vi "SSL Vision Client.vi"() -> ()   [LabVIEW 2016]
uses:
  <vilib>/Utility/tcp.llb/UDP Multicast Read-Only Open.vi
  SSL Detection Robot.ctl
  SSL Detection Ball.ctl
  SSL Detection Frame.ctl
  SSL Geometry Camera Calibration.ctl
panel:
  out "2D Picture":picture
  out "Geometry Camera Calibration":T1
  out "Field Size":T2
  out "Detection Frame":T3
  out "error out":errorcluster
  out "size(s)":i32
  out "unsigned byte array":u8[](array[numeric]) format="%02x"
  in  "Multicast Address:":string="224.5.23.2"
  in  "Multicast Port:":u16=10020
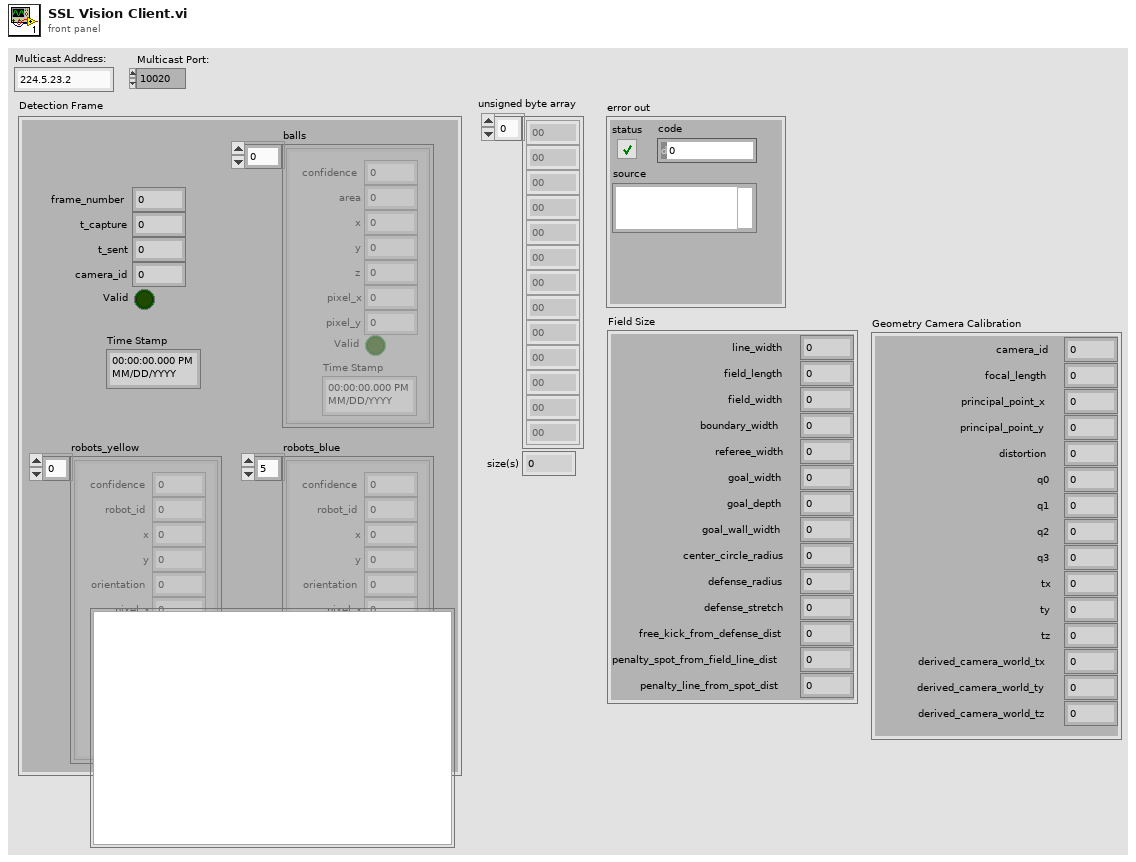
[diagram p1: front panel]
types:
  T1 = typedef "SSL Geometry Camera Calibration.ctl" = cluster{"camera_id":u32, "focal_length":sgl, "principal_point_x":sgl, "principal_point_y":sgl, "distortion":sgl, "q0":sgl, "q1":sgl, "q2":sgl, "q3":sgl, "tx":sgl, "ty":sgl, "tz":sgl, "derived_camera_world_tx":sgl, "derived_camera_world_ty":sgl, "derived_camera_world_tz":sgl}
  T2 = cluster{"line_width":u32, "field_length":u32, "field_width":u32, "boundary_width":u32, "referee_width":u32, "goal_width":u32, "goal_depth":u32, "goal_wall_width":u32, "center_circle_radius":u32, "defense_radius":u32, "defense_stretch":u32, "free_kick_from_defense_dist":u32, "penalty_spot_from_field_line_dist":u32, "penalty_line_from_spot_dist":u32}
  T3 = typedef "SSL Detection Frame.ctl" = cluster{"frame_number":u32, "t_capture":dbl, "t_sent":dbl, "camera_id":u32, "robots_yellow":T4[], "robots_blue":T4[], "balls":T5[], "Valid":bool, "Time Stamp":timestamp}
  T4 = typedef "SSL Detection Robot.ctl" = cluster{"x":dbl, "robot_id":u32, "confidence":sgl, "y":sgl, "orientation":sgl, "pixel_x":sgl, "pixel_y":sgl, "height":sgl, "Valid":bool, "Time Stamp":timestamp}
  T5 = typedef "SSL Detection Ball.ctl" = cluster{"x":sgl, "area":u32, "confidence":sgl, "y":sgl, "z":sgl, "pixel_x":sgl, "pixel_y":sgl, "Valid":bool, "Time Stamp":timestamp}
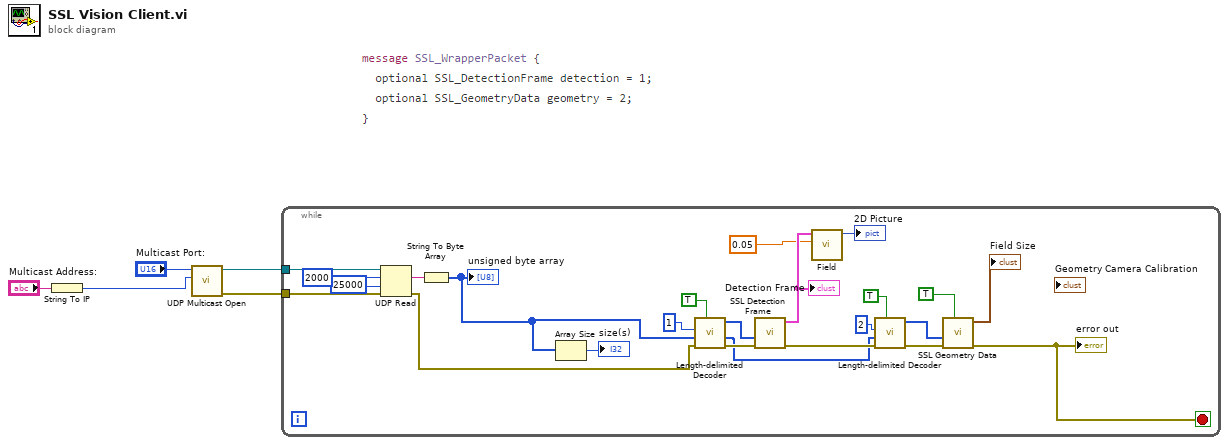
[diagram p0: block diagram]
diagram:
  n1 = String To IP(1:"Multicast Address:") -> (0:w3:u32)
  n2 = call-poly <vilib>:"UDP Multicast Open.vi"("multicast addr"=w3, "port"="Multicast Port:") -> ("error out"=w2:errorcluster, "connection ID"=w1:refnum<k16>)  [unwired: 7 in, 1 out]
  n3 = while {
    tunnel: w2 -> [w29]
    tunnel: w1 -> [w28]
    stop <- w17 stop-if-true
    n4 = UDP Read(connection ID=w28, max size (548)=2000, timeout ms (25000)=25000, 8:w29) -> (data out=w27:string, error out=w20:errorcluster)  [unwired: 3 out]
    n5 = String To Byte Array(string=w27) -> (unsigned byte array=w11:u8[])
    "unsigned byte array" <- w11
    n6 = Array Size(array=w11) -> (size(s)=→"size(s)":i32)
    n7 = call "Length-delimited Decoder.vi"("Optional"=TRUE, "error in (no error)"=w20, "Array"=w11, "Key"=1) -> ("error out"=w22:errorcluster, "array w/ subset deleted"=w14:u8[], "Length-delimited"=w15:u8[])  [unwired: 4 in, 1 out]
    n8 = call "SSL Detection Frame.vi"("error in"=w22, "Array"=w15) -> ("error out"=w21:errorcluster, "Detection Frame"=w8:T3)  [unwired: 8 in]
    "Detection Frame" <- w8
    n9 = call "Field.vi"("Scale mm/pixel"=0.05, "Detection Frame Channel"=w8) -> ("2D Picture"=→"2D Picture":picture)  [unwired: 7 in, 2 out]
    n10 = call "Length-delimited Decoder.vi"("Optional"=TRUE, "error in (no error)"=w21, "Array"=w14, "Key"=2) -> ("error out"=w18:errorcluster, "Length-delimited"=w10:u8[])  [unwired: 4 in, 2 out]
    n11 = call "SSL Geometry Data.vi"("Optional"=TRUE, "error in"=w18, "Array"=w10) -> ("error out"=w17:errorcluster, "Field Size"=→"Field Size":T2)  [unwired: 6 in, 1 out]
    "error out" <- w17
  }
